vi "write1.vi"() -> ()   [LabVIEW 2020]
uses:
  TEST5/LabVIEW Example(8.6)/ControlCAN/ControlCAN.llb/Return Val.ctl
  TEST4/LabVIEW Example(8.6)/ControlCAN/ControlCAN.llb/VCI_CAN_OBJ.ctl
  TEST4/LabVIEW Example(8.6)/ControlCAN/ControlCAN.llb/DevType.ctl
  TEST1/ControlCAN/ControlCAN.llb/VCI_INIT_CONFIG.ctl
  TEST1/ControlCAN/ControlCAN.llb/InitFlag.ctl
  TEST1/ControlCAN/ControlCAN.llb/Fliter.ctl
  TEST1/ControlCAN/ControlCAN.llb/Mode.ctl
  TEST4/LabVIEW Example(8.6)/ControlCAN/ControlCAN.lvlib
panel:
  in  "Len 4":u32=2500 caption="Len(2500)"
  out "Recieve 4":T1[](array[typedef])
  in  "Len 3":u32=2500 caption="Len(2500)"
  out "Recieve 3":T1[](array[typedef])
  in  "Len 2":u32=2500 caption="Len(2500)"
  out "Recieve 2":T1[](array[typedef])
  out "字符串 2":string
  in  "Data 6":string="00 01 02 03 04 05 06 07"
  out "Recieve":T1[](array[typedef])
  in  "Len":u32=2500 caption="Len(2500)"
  in  "选项卡控件":T2(tab)
  in  "位置环KdSet":bool
  in  "位置环的kdread":bool
  in  "位置环kd的值":i32=1000
  in  "位置环KiSet":bool
  in  "位置环的kiread":bool
  in  "ki的值":i32=1000
  in  "kpset":bool
  in  "kpread":bool
  in  "实际位置":bool
  in  "设定位置":bool
  in  "转向电机使能":bool
  in  "停止":bool
  in  "ID":u32=291 format="0x%x"
  in  "转向电机使能：":i32=1000
  in  "位置环：\n     设定位置 2":i32=1000
  in  "kp的值":i32=1000
  out "实际位置":i16
  out "Return Val 2":T3=1 items=["OK"=1, "ERROR1"=0, "ERROR2"=-1]
  # "角度"
  # "角度"
  # "位置环id"
  # "Kp"
  # "Ki"
  # "Kd"
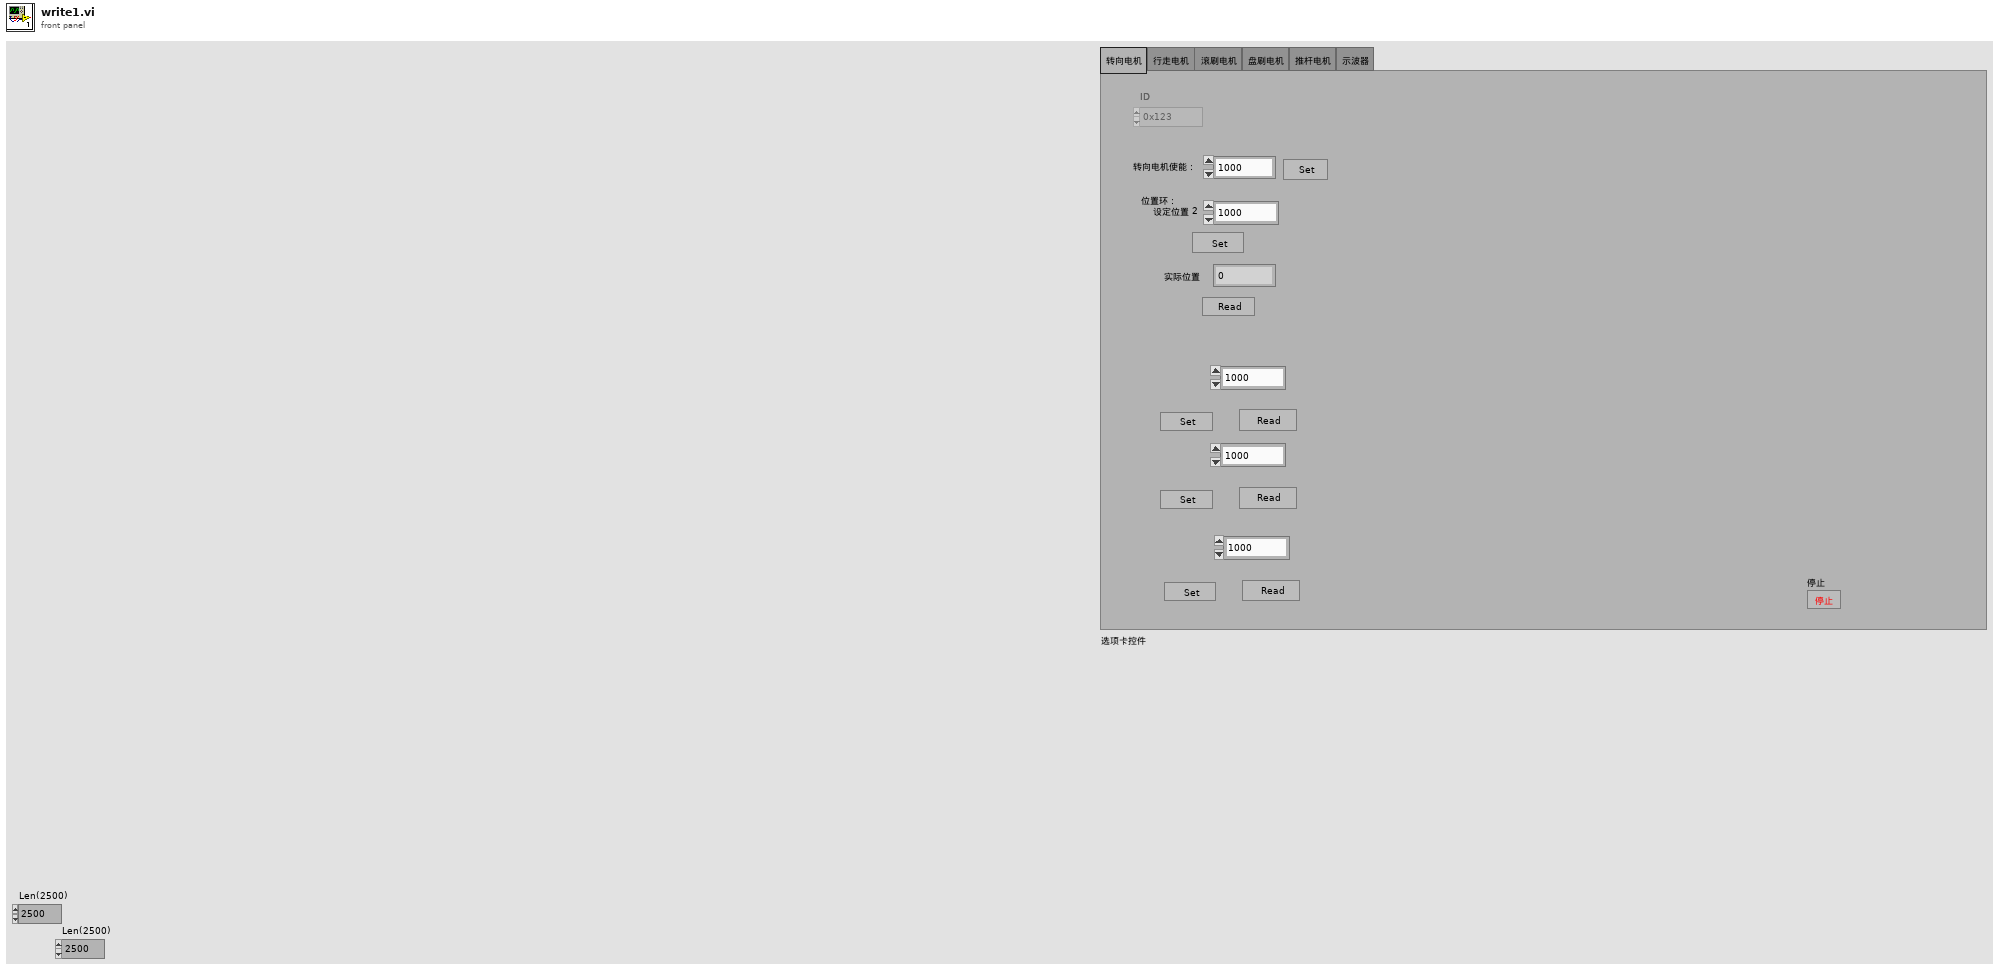
[diagram p1: front panel]
types:
  T1 = typedef "ControlCAN.lvlib/VCI_CAN_OBJ.ctl" = cluster{"ID":u32, "TimeStamp":u32, "TimeFlag":u8, "SendType":u8, "RemoteFlag":u8, "ExternFlag":u8, "DataLen":u8, "Data":u8[], "Reserved":u8[]}
  T2 = enum32{"转向电机", "行走电机", "滚刷电机", "盘刷电机", "推杆电机", "示波器"}
  T3 = typedef "ControlCAN.lvlib/Return Val.ctl" = i32
  T4 = typedef "ControlCAN.lvlib/VCI_INIT_CONFIG.ctl" = cluster{"AccCode":u32, "AccMask":u32, "InitFlag":T5, "Fliter":T6, "Timing0":u8, "Timing1":u8, "Mode":T7}
  T5 = typedef "ControlCAN.lvlib/InitFlag.ctl" = u32
  T6 = typedef "ControlCAN.lvlib/Fliter.ctl" = u8
  T7 = typedef "ControlCAN.lvlib/Mode.ctl" = u8
  T8 = typedef "ControlCAN.lvlib/DevType.ctl" = u32
  T9 = cluster{"Recieve 2[0]":T1, "Recieve 2[1]":T1, "Recieve 2[2]":T1, "Recieve 2[3]":T1, "Recieve 2[4]":T1, "Recieve 2[5]":T1, "Recieve 2[6]":T1, "Recieve 2[7]":T1, "Recieve 2[8]":T1}
  T10 = cluster{"Data[0]":u8, "Data[1]":u8, "Data[2]":u8, "Data[3]":u8, "Data[4]":u8, "Data[5]":u8, "Data[6]":u8, "Data[7]":u8, "Data[8]":u8}
  T11 = cluster{"Recieve[0]":T1, "Recieve[1]":T1, "Recieve[2]":T1, "Recieve[3]":T1, "Recieve[4]":T1, "Recieve[5]":T1, "Recieve[6]":T1, "Recieve[7]":T1, "Recieve[8]":T1}
  T12 = cluster{"Recieve 3[0]":T1, "Recieve 3[1]":T1, "Recieve 3[2]":T1, "Recieve 3[3]":T1, "Recieve 3[4]":T1, "Recieve 3[5]":T1, "Recieve 3[6]":T1, "Recieve 3[7]":T1, "Recieve 3[8]":T1}
  T13 = cluster{"Recieve 4[0]":T1, "Recieve 4[1]":T1, "Recieve 4[2]":T1, "Recieve 4[3]":T1, "Recieve 4[4]":T1, "Recieve 4[5]":T1, "Recieve 4[6]":T1, "Recieve 4[7]":T1, "Recieve 4[8]":T1}
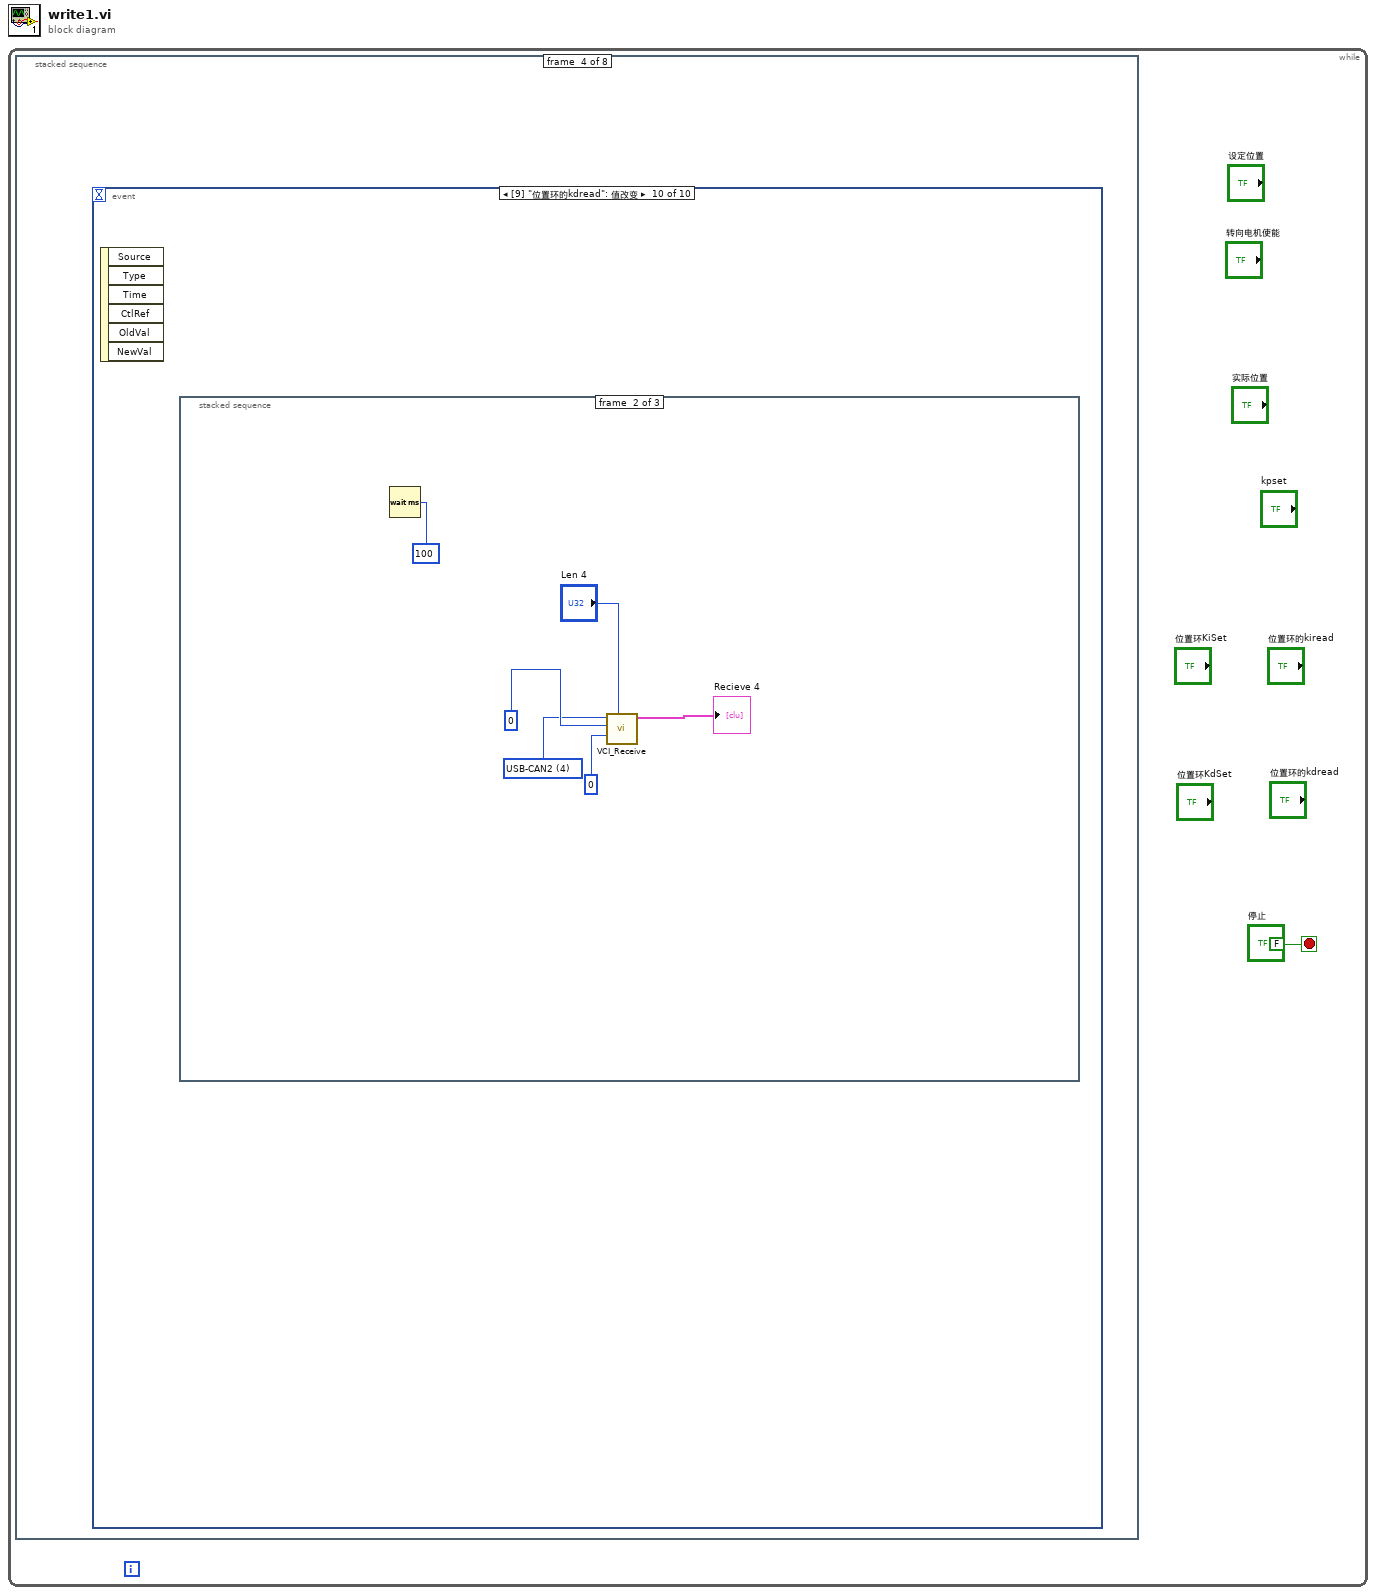
[diagram p0: block diagram]
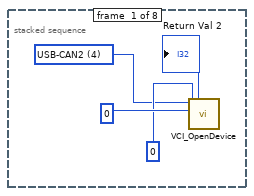
[diagram p2: hidden frame]
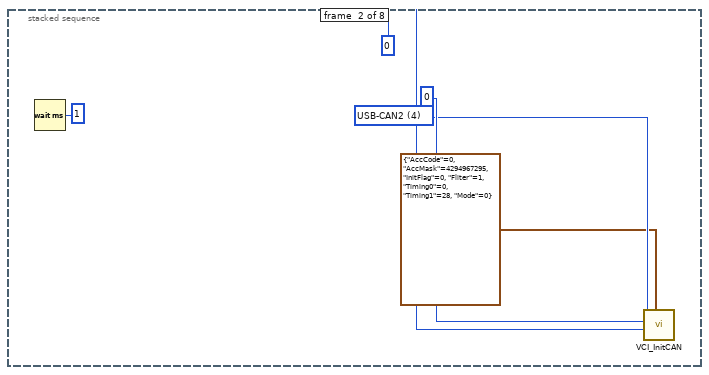
[diagram p3: hidden frame]
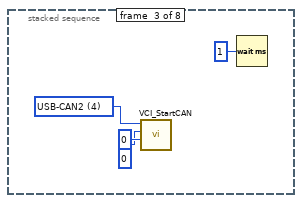
[diagram p4: hidden frame]
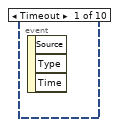
[diagram p5: hidden frame]
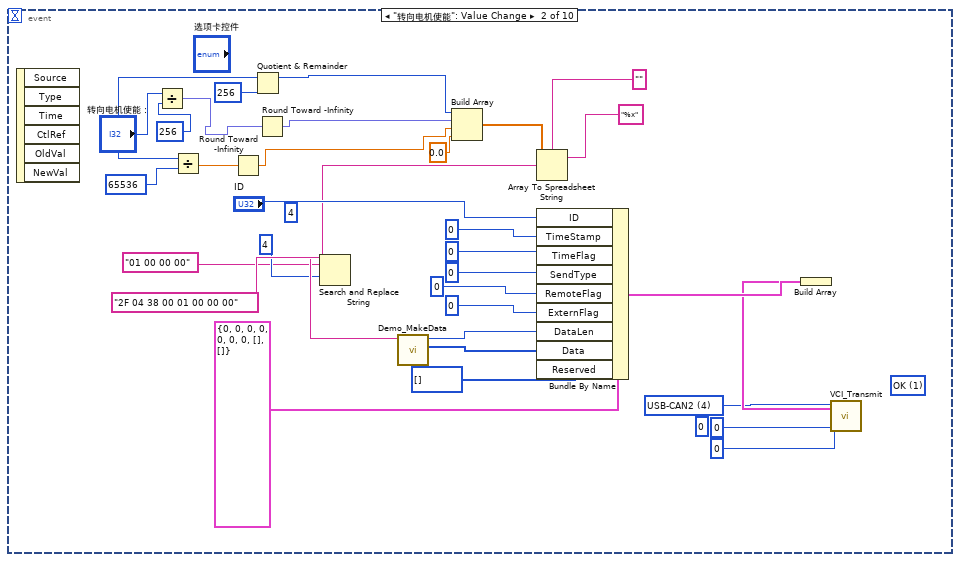
[diagram p6: hidden frame]
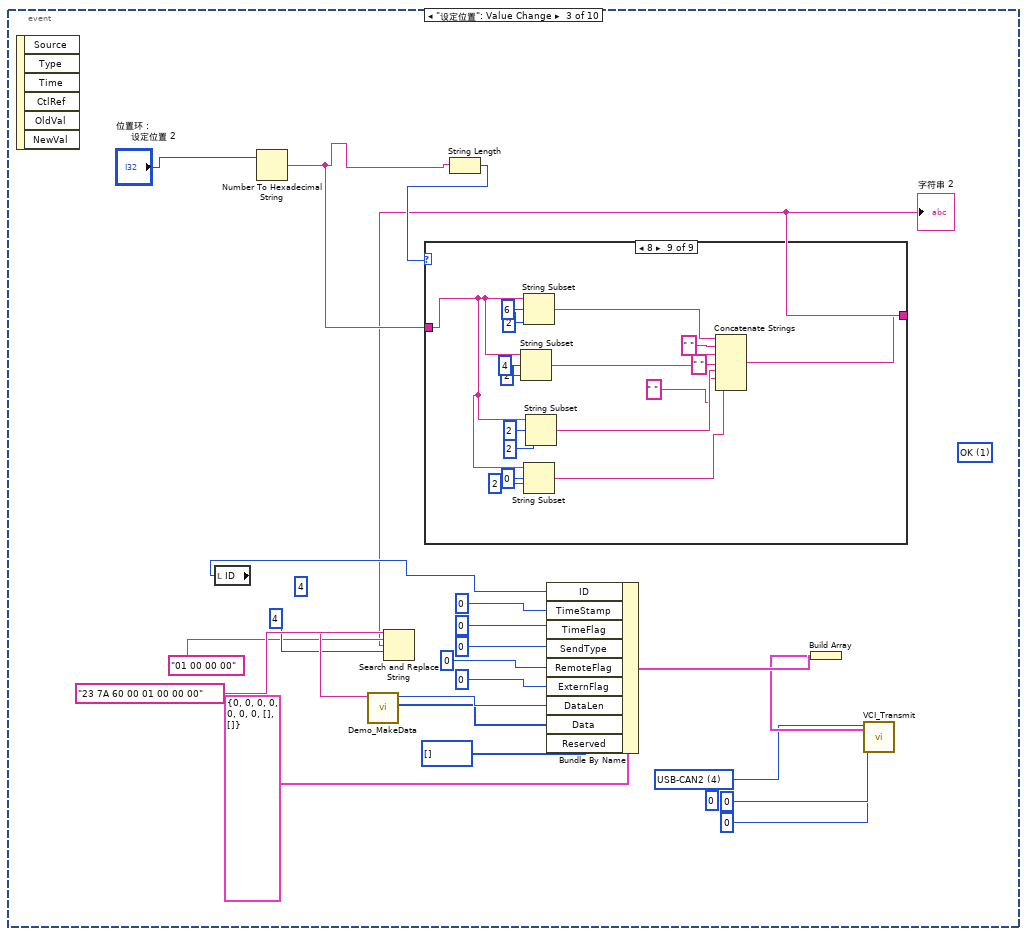
[diagram p7: hidden frame]
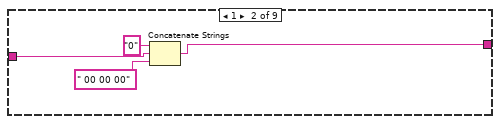
[diagram p9: hidden frame]
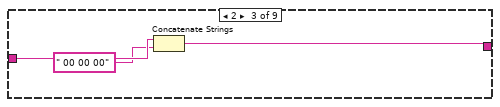
[diagram p10: hidden frame]
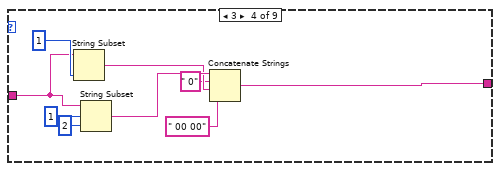
[diagram p11: hidden frame]
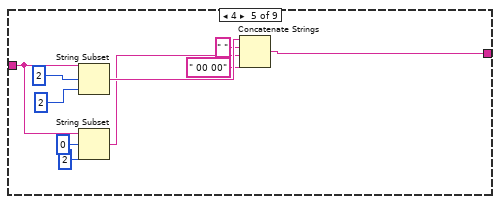
[diagram p12: hidden frame]
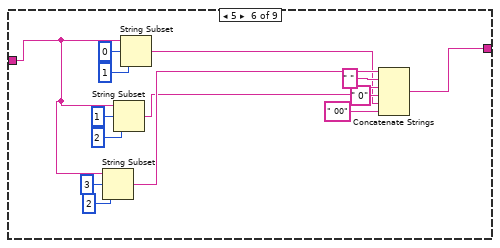
[diagram p13: hidden frame]
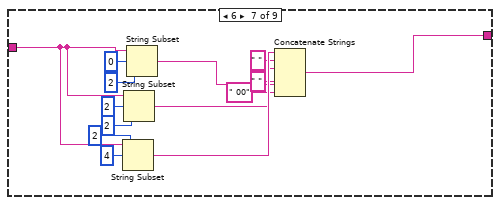
[diagram p14: hidden frame]
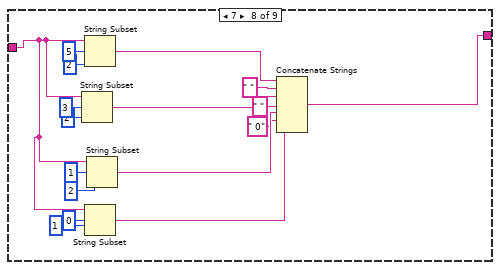
[diagram p15: hidden frame]
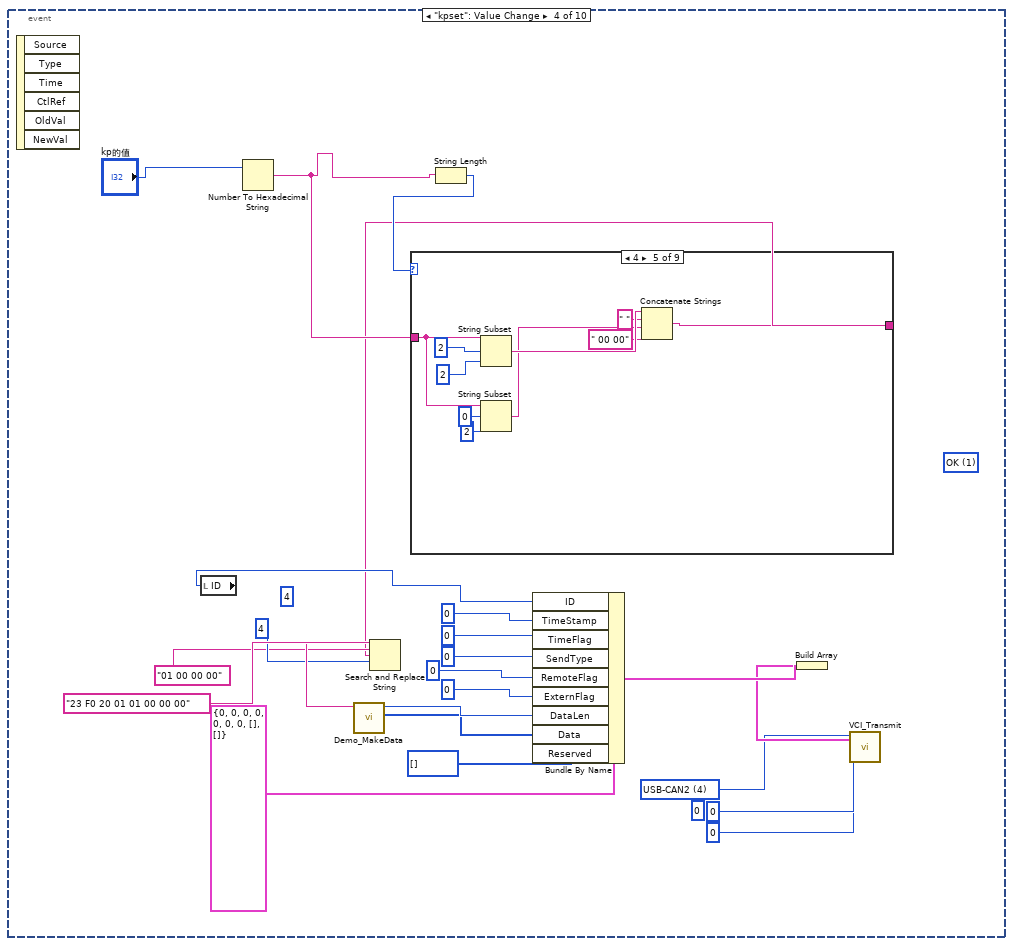
[diagram p16: hidden frame]
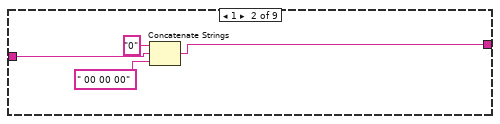
[diagram p18: hidden frame]
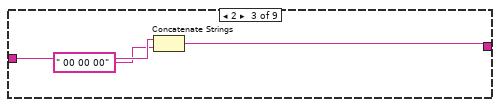
[diagram p19: hidden frame]
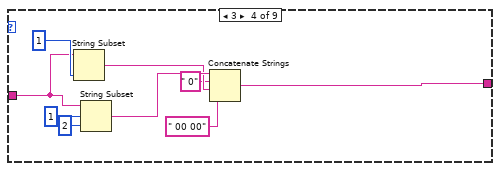
[diagram p20: hidden frame]
diagram:
  n1 = while {
    stop <- FALSE stop-if-true
    n2 = stacked-sequence {
      frame #0 {
        w2 = T8 4 items=["USB-CAN"=3, "USB-CAN2"=4] ("DevType")
        n3 = call "VCI_OpenDevice.vi"("Reserved"=u32 0, "DevIndex"=u32 0, "DevType"=w2) -> ("Return Val"=→"Return Val 2":T3)  [unwired: 7 in, 1 out]
      }
      frame #1 {
        w8 = T8 4 items=["USB-CAN"=3, "USB-CAN2"=4] ("DevType")
        n4 = Wait (ms)(milliseconds to wait=u32 1 ("等待时间（毫秒）")) -> ()  [unwired: 1 out]
        n5 = call "VCI_InitCAN.vi"("VCI_INIT_CONFIG"=T4 {"AccCode"=0, "AccMask"=4294967295, "InitFlag"=0, "Fliter"=1, "Timing0"=0, "Timing1"=28, "Mode"=0}, "CANIndex"=u32 0, "DevIndex"=u32 0, "DevType"=w8) -> ()  [unwired: 6 in, 2 out]
      }
      frame #2 {
        w12 = T8 4 items=["USB-CAN"=3, "USB-CAN2"=4] ("DevType")
        n6 = call "VCI_StartCAN.vi"("CANIndex"=u32 0, "DevIndex"=u32 0, "DevType"=w12) -> ()  [unwired: 7 in, 2 out]
        n7 = Wait (ms)(milliseconds to wait=u32 1 ("等待时间（毫秒）")) -> ()  [unwired: 1 out]
      }
      frame #3 {
        n8 = event shown="[9] \"位置环的kdread\": 值改变" {
          selector: _ -> [_ _ _ _ _ _ _ _ _ _]
          dyn-events: _ -> [_ _ _ _ _ _ _ _ _ _]
          timeout: _ -> [_ _ _ _ _ _ _ _ _ _]
          event Timeout {
            n9 = event-data() -> ()  [unwired: 1 in, 3 out]
          }
          event "转向电机使能": Value Change {
            (unwired) 4 ("替换数量")
            (unwired) T3 1 items=["OK"=1, "ERROR1"=0, "ERROR2"=-1] ("Return Val")
            (unwired) u32 0 ("CANIndex")
            w36 = T8 4 items=["USB-CAN"=3, "USB-CAN2"=4] ("DevType")
            n10 = event-data() -> ()  [unwired: 1 in, 6 out]
            n11 = Divide ("除")(x="转向电机使能：", y=256) -> (x/y=w20:fxp<+/-,32,16>)
            n12 = Divide(x="转向电机使能：", y=65536) -> (x/y=w17:dbl)
            n13 = Round Toward -Infinity(1:w17) -> (0:w16:dbl)
            n14 = Quotient & Remainder(x="转向电机使能：", y=256) -> (x-y*floor(x/y)=w19:i32)  [unwired: 1 out]
            n15 = Round Toward -Infinity(1:w20) -> (0:w18:fxp<+/-,16,16>)
            n16 = Build Array(w19, w18, w16, 0.0 ("元素")) -> (w25:dbl[])
            n17 = Array To Spreadsheet String(delimiter (Tab)="" ("分隔符(Tab)"), array=w25, 3:"%x" ("格式字符串")) -> (spreadsheet string=w26:string)
            n18 = Search and Replace String(input string="2F 04 38 00 01 00 00 00" ("Data 2"), search string="01 00 00 00" ("Data 4"), replace string=w26, offset=4 ("偏移量(0)")) -> (result string=w31:string)  [unwired: 4 in, 3 out]
            n19 = call "Demo_MakeData.vi"("DataString"=w31) -> ("Data"=w43:u8[], "DataLen"=w44:u8)  [unwired: 9 out]
            n20 = Bundle By Name(cluster=T1 {"ID"=0, "TimeStamp"=0, "TimeFlag"=0, "SendType"=0, "RemoteFlag"=0, "ExternFlag"=0, "DataLen"=0, "Data"=[], "Reserved"=[]} ("Send"), "ID"="ID", "TimeStamp"=u32 0, "TimeFlag"=u8 0, "SendType"=u8 0, "RemoteFlag"=u8 0, "ExternFlag"=u8 0, "DataLen"=w44, "Data"=w43, "Reserved"=u8[] []) -> (w46:T1)
            n21 = Build Array(w46) -> (w45:T1[])
            n22 = call "VCI_Transmit.vi"("Buffer"=w45, "CANIndex"=u32 0, "DevIndex"=u32 0, "DevType"=w36) -> ()  [unwired: 6 in, 2 out]
          }
          event "设定位置": Value Change {
            (unwired) 4 ("替换数量")
            (unwired) T3 1 items=["OK"=1, "ERROR1"=0, "ERROR2"=-1] ("Return Val")
            (unwired) u32 0 ("CANIndex")
            w61 = T8 4 items=["USB-CAN"=3, "USB-CAN2"=4] ("DevType")
            n23 = event-data() -> ()  [unwired: 1 in, 6 out]
            n24 = local read "ID"() -> (w53:u32)
            n25 = Number To Hexadecimal String(2:"位置环：\n     设定位置 2") -> (0:w49:string)  [unwired: 1 in]
            n26 = String Length(string=w49) -> (length=w50:i32)
            n27 = case shown="8" w50 {
              tunnel: w49 -> [w71 w74 w77 w84 w93 w107 w120 w136 w146]
              tunnel: [w71 w73 w78 w79 w97 w104 w125 w126 w145] -> w48
              frame 0, Default {
              }
              frame 1 {
                n28 = Concatenate Strings("0" ("字符串"), w74, " 00 00 00" ("字符串")) -> (w73:string)
              }
              frame 2 {
                n29 = Concatenate Strings(w77, " 00 00 00" ("字符串")) -> (w78:string)
              }
              frame 3 {
                n30 = String Subset(string=w84, length (rest)=1 ("长度（剩余）")) -> (substring=w82:string)  [unwired: 1 in]
                n31 = String Subset(string=w84, offset (0)=1 ("偏移量(0)"), length (rest)=2 ("长度（剩余）")) -> (substring=w83:string)
                n32 = Concatenate Strings(w83, " 0" ("字符串"), w82, " 00 00" ("字符串")) -> (w79:string)
              }
              frame 4 {
                n33 = String Subset(string=w93, offset (0)=2 ("偏移量(0)"), length (rest)=2 ("长度（剩余）")) -> (substring=w94:string)
                n34 = String Subset(string=w93, offset (0)=0 ("偏移量(0)"), length (rest)=2 ("长度（剩余）")) -> (substring=w89:string)
                n35 = Concatenate Strings(w94, " " ("字符串"), w89, " 00 00" ("字符串")) -> (w97:string)
              }
              frame 5 {
                n36 = String Subset(string=w107, offset (0)=3 ("偏移量(0)"), length (rest)=2 ("长度（剩余）")) -> (substring=w103:string)
                n37 = String Subset(string=w107, offset (0)=1 ("偏移量(0)"), length (rest)=2 ("长度（剩余）")) -> (substring=w101:string)
                n38 = String Subset(string=w107, offset (0)=0 ("偏移量(0)"), length (rest)=1 ("长度（剩余）")) -> (substring=w99:string)
                n39 = Concatenate Strings(w103, " " ("字符串"), w101, " 0" ("字符串"), w99, " 00" ("字符串")) -> (w104:string)
              }
              frame 6 {
                n40 = String Subset(string=w120, offset (0)=4 ("偏移量(0)"), length (rest)=2 ("长度（剩余）")) -> (substring=w117:string)
                n41 = String Subset(string=w120, offset (0)=2 ("偏移量(0)"), length (rest)=2 ("长度（剩余）")) -> (substring=w115:string)
                n42 = String Subset(string=w120, offset (0)=0 ("偏移量(0)"), length (rest)=2 ("长度（剩余）")) -> (substring=w113:string)
                n43 = Concatenate Strings(w117, " " ("字符串"), w115, " " ("字符串"), w113, " 00" ("字符串")) -> (w125:string)
              }
              frame 7 {
                n44 = String Subset(string=w136, offset (0)=3 ("偏移量(0)"), length (rest)=2 ("长度（剩余）")) -> (substring=w131:string)
                n45 = String Subset(string=w136, offset (0)=5 ("偏移量(0)"), length (rest)=2 ("长度（剩余）")) -> (substring=w133:string)
                n46 = String Subset(string=w136, offset (0)=0 ("偏移量(0)"), length (rest)=1 ("长度（剩余）")) -> (substring=w127:string)
                n47 = String Subset(string=w136, offset (0)=1 ("偏移量(0)"), length (rest)=2 ("长度（剩余）")) -> (substring=w129:string)
                n48 = Concatenate Strings(w133, " " ("字符串"), w131, " " ("字符串"), w129, " 0" ("字符串"), w127) -> (w126:string)
              }
              frame 8 {
                n49 = String Subset(string=w146, offset (0)=4 ("偏移量(0)"), length (rest)=2 ("长度（剩余）")) -> (substring=w149:string)
                n50 = String Subset(string=w146, offset (0)=6 ("偏移量(0)"), length (rest)=2 ("长度（剩余）")) -> (substring=w151:string)
                n51 = String Subset(string=w146, offset (0)=0 ("偏移量(0)"), length (rest)=2 ("长度（剩余）")) -> (substring=w143:string)
                n52 = String Subset(string=w146, offset (0)=2 ("偏移量(0)"), length (rest)=2 ("长度（剩余）")) -> (substring=w147:string)
                n53 = Concatenate Strings(w151, " " ("字符串"), w149, " " ("字符串"), w147, " " ("字符串"), w143) -> (w145:string)
              }
            }
            "字符串 2" <- w48
            n54 = Search and Replace String(input string="23 7A 60 00 01 00 00 00" ("Data 3"), search string="01 00 00 00" ("Data 5"), replace string=w48, offset=4 ("偏移量(0)")) -> (result string=w56:string)  [unwired: 4 in, 3 out]
            n55 = call "Demo_MakeData.vi"("DataString"=w56) -> ("Data"=w52:u8[], "DataLen"=w67:u8)  [unwired: 9 out]
            n56 = Bundle By Name(cluster=T1 {"ID"=0, "TimeStamp"=0, "TimeFlag"=0, "SendType"=0, "RemoteFlag"=0, "ExternFlag"=0, "DataLen"=0, "Data"=[], "Reserved"=[]} ("Send"), "ID"=w53, "TimeStamp"=u32 0, "TimeFlag"=u8 0, "SendType"=u8 0, "RemoteFlag"=u8 0, "ExternFlag"=u8 0, "DataLen"=w67, "Data"=w52, "Reserved"=u8[] []) -> (w69:T1)
            n57 = Build Array(w69) -> (w68:T1[])
            n58 = call "VCI_Transmit.vi"("Buffer"=w68, "CANIndex"=u32 0, "DevIndex"=u32 0, "DevType"=w61) -> ()  [unwired: 6 in, 2 out]
          }
          event "kpset": Value Change {
            (unwired) 4 ("替换数量")
            (unwired) T3 1 items=["OK"=1, "ERROR1"=0, "ERROR2"=-1] ("Return Val")
            (unwired) u32 0 ("CANIndex")
            w173 = T8 4 items=["USB-CAN"=3, "USB-CAN2"=4] ("DevType")
            n59 = event-data() -> ()  [unwired: 1 in, 6 out]
            n60 = local read "ID"() -> (w165:u32)
            n61 = Number To Hexadecimal String(2:"kp的值") -> (0:w162:string)  [unwired: 1 in]
            n62 = String Length(string=w162) -> (length=w163:i32)
            n63 = case shown="4" w163 {
              tunnel: w162 -> [w183 w186 w189 w196 w205 w219 w232 w248 w258]
              tunnel: [w183 w185 w190 w191 w209 w216 w237 w238 w257] -> w160
              frame 0, Default {
              }
              frame 1 {
                n64 = Concatenate Strings("0" ("字符串"), w186, " 00 00 00" ("字符串")) -> (w185:string)
              }
              frame 2 {
                n65 = Concatenate Strings(w189, " 00 00 00" ("字符串")) -> (w190:string)
              }
              frame 3 {
                n66 = String Subset(string=w196, length (rest)=1 ("长度（剩余）")) -> (substring=w194:string)  [unwired: 1 in]
                n67 = String Subset(string=w196, offset (0)=1 ("偏移量(0)"), length (rest)=2 ("长度（剩余）")) -> (substring=w195:string)
                n68 = Concatenate Strings(w195, " 0" ("字符串"), w194, " 00 00" ("字符串")) -> (w191:string)
              }
              frame 4 {
                n69 = String Subset(string=w205, offset (0)=2 ("偏移量(0)"), length (rest)=2 ("长度（剩余）")) -> (substring=w206:string)
                n70 = String Subset(string=w205, offset (0)=0 ("偏移量(0)"), length (rest)=2 ("长度（剩余）")) -> (substring=w201:string)
                n71 = Concatenate Strings(w206, " " ("字符串"), w201, " 00 00" ("字符串")) -> (w209:string)
              }
              frame 5 {
                n72 = String Subset(string=w219, offset (0)=3 ("偏移量(0)"), length (rest)=2 ("长度（剩余）")) -> (substring=w215:string)
                n73 = String Subset(string=w219, offset (0)=1 ("偏移量(0)"), length (rest)=2 ("长度（剩余）")) -> (substring=w213:string)
                n74 = String Subset(string=w219, offset (0)=0 ("偏移量(0)"), length (rest)=1 ("长度（剩余）")) -> (substring=w211:string)
                n75 = Concatenate Strings(w215, " " ("字符串"), w213, " 0" ("字符串"), w211, " 00" ("字符串")) -> (w216:string)
              }
              frame 6 {
                n76 = String Subset(string=w232, offset (0)=4 ("偏移量(0)"), length (rest)=2 ("长度（剩余）")) -> (substring=w229:string)
                n77 = String Subset(string=w232, offset (0)=2 ("偏移量(0)"), length (rest)=2 ("长度（剩余）")) -> (substring=w227:string)
                n78 = String Subset(string=w232, offset (0)=0 ("偏移量(0)"), length (rest)=2 ("长度（剩余）")) -> (substring=w225:string)
                n79 = Concatenate Strings(w229, " " ("字符串"), w227, " " ("字符串"), w225, " 00" ("字符串")) -> (w237:string)
              }
              frame 7 {
                n80 = String Subset(string=w248, offset (0)=3 ("偏移量(0)"), length (rest)=2 ("长度（剩余）")) -> (substring=w243:string)
                n81 = String Subset(string=w248, offset (0)=5 ("偏移量(0)"), length (rest)=2 ("长度（剩余）")) -> (substring=w245:string)
                n82 = String Subset(string=w248, offset (0)=0 ("偏移量(0)"), length (rest)=1 ("长度（剩余）")) -> (substring=w239:string)
                n83 = String Subset(string=w248, offset (0)=1 ("偏移量(0)"), length (rest)=2 ("长度（剩余）")) -> (substring=w241:string)
                n84 = Concatenate Strings(w245, " " ("字符串"), w243, " " ("字符串"), w241, " 0" ("字符串"), w239) -> (w238:string)
              }
              frame 8 {
                n85 = String Subset(string=w258, offset (0)=4 ("偏移量(0)"), length (rest)=2 ("长度（剩余）")) -> (substring=w261:string)
                n86 = String Subset(string=w258, offset (0)=6 ("偏移量(0)"), length (rest)=2 ("长度（剩余）")) -> (substring=w263:string)
                n87 = String Subset(string=w258, offset (0)=0 ("偏移量(0)"), length (rest)=2 ("长度（剩余）")) -> (substring=w255:string)
                n88 = String Subset(string=w258, offset (0)=2 ("偏移量(0)"), length (rest)=2 ("长度（剩余）")) -> (substring=w259:string)
                n89 = Concatenate Strings(w263, " " ("字符串"), w261, " " ("字符串"), w259, " " ("字符串"), w255) -> (w257:string)
              }
            }
            n90 = Search and Replace String(input string="23 F0 20 01 01 00 00 00" ("Data 3"), search string="01 00 00 00" ("Data 5"), replace string=w160, offset=4 ("偏移量(0)")) -> (result string=w168:string)  [unwired: 4 in, 3 out]
            n91 = call "Demo_MakeData.vi"("DataString"=w168) -> ("Data"=w164:u8[], "DataLen"=w179:u8)  [unwired: 9 out]
            n92 = Bundle By Name(cluster=T1 {"ID"=0, "TimeStamp"=0, "TimeFlag"=0, "SendType"=0, "RemoteFlag"=0, "ExternFlag"=0, "DataLen"=0, "Data"=[], "Reserved"=[]} ("Send"), "ID"=w165, "TimeStamp"=u32 0, "TimeFlag"=u8 0, "SendType"=u8 0, "RemoteFlag"=u8 0, "ExternFlag"=u8 0, "DataLen"=w179, "Data"=w164, "Reserved"=u8[] []) -> (w181:T1)
            n93 = Build Array(w181) -> (w180:T1[])
            n94 = call "VCI_Transmit.vi"("Buffer"=w180, "CANIndex"=u32 0, "DevIndex"=u32 0, "DevType"=w173) -> ()  [unwired: 6 in, 2 out]
          }
          event "kpread": Value Change {
            n95 = event-data() -> ()  [unwired: 1 in, 6 out]
            n96 = stacked-sequence {
              frame #0 {
                (unwired) u32 0 ("CANIndex")
                w278 = T8 4 items=["USB-CAN"=3, "USB-CAN2"=4] ("DevType")
                n97 = local read "ID"() -> (w273:u32)
                n98 = call "Demo_MakeData.vi"("DataString"="40 F0 20 01 00 00 00 00" ("Data 7")) -> ("Data"=w284:u8[], "DataLen"=w285:u8)  [unwired: 9 out]
                n99 = Bundle By Name(cluster=T1 {"ID"=0, "TimeStamp"=0, "TimeFlag"=0, "SendType"=0, "RemoteFlag"=0, "ExternFlag"=0, "DataLen"=0, "Data"=[], "Reserved"=[]} ("Send"), "ID"=w273, "TimeStamp"=u32 0, "TimeFlag"=u8 0, "SendType"=u8 0, "RemoteFlag"=u8 0, "ExternFlag"=u8 0, "DataLen"=w285, "Data"=w284, "Reserved"=u8[] []) -> (w287:T1)
                n100 = Build Array(w287) -> (w286:T1[])
                n101 = call "VCI_Transmit.vi"("Buffer"=w286, "CANIndex"=u32 0, "DevIndex"=u32 0, "DevType"=w278) -> ()  [unwired: 6 in, 2 out]
              }
              frame #1 {
                w288 = T8 4 items=["USB-CAN"=3, "USB-CAN2"=4] ("DevType")
                n102 = Wait (ms)(milliseconds to wait=u32 100 ("等待时间（毫秒）")) -> ()  [unwired: 1 out]
                n103 = call "VCI_Receive.vi"("Len"="Len 2", "CANIndex"=u32 0, "DevIndex"=u32 0, "DevType"=w288) -> ("Recieve"=→"Recieve 2":T1[])  [unwired: 6 in, 1 out]
              }
              frame #2 {
                n104 = local read "Recieve 2"() -> (w310:T1[])
                n105 = Array To Cluster(array=w310) -> (cluster=w309:T9)
                n106 = Unbundle By Name(w309) -> ("Recieve 2[0].Data"=w308:u8[])
                n107 = Array To Cluster(array=w308) -> (cluster=w307:T10)
                n108 = Unbundle By Name(w307) -> ("Data[6]"=w302:u8)
                n109 = Unbundle By Name(w307) -> ("Data[7]"=w301:u8)
                n110 = Unbundle By Name(w307) -> ("Data[5]"=w306:u8)
                n111 = Unbundle By Name(w307) -> ("Data[4]"=w303:u8)
                n112 = Multiply(x=w301, y=16777216) -> (x*y=w297:i32)
                n113 = Multiply(x=w302, y=65536) -> (x*y=w298:i32)
                n114 = Multiply(x=w306, y=256.0) -> (x*y=w304:dbl)
                n115 = Add(x=w303, y=w304) -> (x+y=w296:dbl)
                n116 = Add(x=w298, y=w297) -> (x+y=w295:i32)
                n117 = Add(x=w296, y=w295) -> (x+y=→"实际位置":dbl)
              }
            }
          }
          event "实际位置": Value Change {
            n118 = event-data() -> ()  [unwired: 1 in, 6 out]
            n119 = stacked-sequence {
              frame #0 {
                (unwired) u32 0 ("CANIndex")
                w317 = T8 4 items=["USB-CAN"=3, "USB-CAN2"=4] ("DevType")
                n120 = local read "ID"() -> (w312:u32)
                n121 = call "Demo_MakeData.vi"("DataString"="Data 6") -> ("Data"=w323:u8[], "DataLen"=w324:u8)  [unwired: 9 out]
                n122 = Bundle By Name(cluster=T1 {"ID"=0, "TimeStamp"=0, "TimeFlag"=0, "SendType"=0, "RemoteFlag"=0, "ExternFlag"=0, "DataLen"=0, "Data"=[], "Reserved"=[]} ("Send"), "ID"=w312, "TimeStamp"=u32 0, "TimeFlag"=u8 0, "SendType"=u8 0, "RemoteFlag"=u8 0, "ExternFlag"=u8 0, "DataLen"=w324, "Data"=w323, "Reserved"=u8[] []) -> (w326:T1)
                n123 = Build Array(w326) -> (w325:T1[])
                n124 = call "VCI_Transmit.vi"("Buffer"=w325, "CANIndex"=u32 0, "DevIndex"=u32 0, "DevType"=w317) -> ()  [unwired: 6 in, 2 out]
              }
              frame #1 {
                w327 = T8 4 items=["USB-CAN"=3, "USB-CAN2"=4] ("DevType")
                n125 = Wait (ms)(milliseconds to wait=u32 100 ("等待时间（毫秒）")) -> ()  [unwired: 1 out]
                n126 = call "VCI_Receive.vi"("Len"="Len", "CANIndex"=u32 0, "DevIndex"=u32 0, "DevType"=w327) -> ("Recieve"=→"Recieve":T1[])  [unwired: 6 in, 1 out]
              }
              frame #2 {
                n127 = local read "Recieve"() -> (w349:T1[])
                n128 = Array To Cluster(array=w349) -> (cluster=w348:T11)
                n129 = Unbundle By Name(w348) -> ("Recieve[0].Data"=w347:u8[])
                n130 = Array To Cluster(array=w347) -> (cluster=w346:T10)
                n131 = Unbundle By Name(w346) -> ("Data[6]"=w341:u8)
                n132 = Unbundle By Name(w346) -> ("Data[7]"=w340:u8)
                n133 = Unbundle By Name(w346) -> ("Data[5]"=w345:u8)
                n134 = Unbundle By Name(w346) -> ("Data[4]"=w342:u8)
                n135 = Multiply(x=w340, y=16777216) -> (x*y=w336:i32)
                n136 = Multiply(x=w341, y=65536) -> (x*y=w337:i32)
                n137 = Multiply(x=w345, y=256.0) -> (x*y=w343:dbl)
                n138 = Add(x=w342, y=w343) -> (x+y=w335:dbl)
                n139 = Add(x=w337, y=w336) -> (x+y=w334:i32)
                n140 = Add(x=w335, y=w334) -> (x+y=w333:dbl)
                n141 = local write "kp的值"(w333) -> ()
              }
            }
          }
          event "位置环KiSet": Value Change {
            (unwired) 4 ("替换数量")
            (unwired) u32 0 ("CANIndex")
            w363 = T8 4 items=["USB-CAN"=3, "USB-CAN2"=4] ("DevType")
            n142 = event-data() -> ()  [unwired: 1 in, 6 out]
            n143 = local read "ID"() -> (w355:u32)
            n144 = Number To Hexadecimal String(2:"ki的值") -> (0:w352:string)  [unwired: 1 in]
            n145 = String Length(string=w352) -> (length=w353:i32)
            n146 = case shown="4" w353 {
              tunnel: w352 -> [w373 w376 w379 w386 w395 w409 w422 w438 w448]
              tunnel: [w373 w375 w380 w381 w399 w406 w427 w428 w447] -> w351
              frame 0, Default {
              }
              frame 1 {
                n147 = Concatenate Strings("0" ("字符串"), w376, " 00 00 00" ("字符串")) -> (w375:string)
              }
              frame 2 {
                n148 = Concatenate Strings(w379, " 00 00 00" ("字符串")) -> (w380:string)
              }
              frame 3 {
                n149 = String Subset(string=w386, length (rest)=1 ("长度（剩余）")) -> (substring=w384:string)  [unwired: 1 in]
                n150 = String Subset(string=w386, offset (0)=1 ("偏移量(0)"), length (rest)=2 ("长度（剩余）")) -> (substring=w385:string)
                n151 = Concatenate Strings(w385, " 0" ("字符串"), w384, " 00 00" ("字符串")) -> (w381:string)
              }
              frame 4 {
                n152 = String Subset(string=w395, offset (0)=2 ("偏移量(0)"), length (rest)=2 ("长度（剩余）")) -> (substring=w396:string)
                n153 = String Subset(string=w395, offset (0)=0 ("偏移量(0)"), length (rest)=2 ("长度（剩余）")) -> (substring=w391:string)
                n154 = Concatenate Strings(w396, " " ("字符串"), w391, " 00 00" ("字符串")) -> (w399:string)
              }
              frame 5 {
                n155 = String Subset(string=w409, offset (0)=3 ("偏移量(0)"), length (rest)=2 ("长度（剩余）")) -> (substring=w405:string)
                n156 = String Subset(string=w409, offset (0)=1 ("偏移量(0)"), length (rest)=2 ("长度（剩余）")) -> (substring=w403:string)
                n157 = String Subset(string=w409, offset (0)=0 ("偏移量(0)"), length (rest)=1 ("长度（剩余）")) -> (substring=w401:string)
                n158 = Concatenate Strings(w405, " " ("字符串"), w403, " 0" ("字符串"), w401, " 00" ("字符串")) -> (w406:string)
              }
              frame 6 {
                n159 = String Subset(string=w422, offset (0)=4 ("偏移量(0)"), length (rest)=2 ("长度（剩余）")) -> (substring=w419:string)
                n160 = String Subset(string=w422, offset (0)=2 ("偏移量(0)"), length (rest)=2 ("长度（剩余）")) -> (substring=w417:string)
                n161 = String Subset(string=w422, offset (0)=0 ("偏移量(0)"), length (rest)=2 ("长度（剩余）")) -> (substring=w415:string)
                n162 = Concatenate Strings(w419, " " ("字符串"), w417, " " ("字符串"), w415, " 00" ("字符串")) -> (w427:string)
              }
              frame 7 {
                n163 = String Subset(string=w438, offset (0)=3 ("偏移量(0)"), length (rest)=2 ("长度（剩余）")) -> (substring=w433:string)
                n164 = String Subset(string=w438, offset (0)=5 ("偏移量(0)"), length (rest)=2 ("长度（剩余）")) -> (substring=w435:string)
                n165 = String Subset(string=w438, offset (0)=0 ("偏移量(0)"), length (rest)=1 ("长度（剩余）")) -> (substring=w429:string)
                n166 = String Subset(string=w438, offset (0)=1 ("偏移量(0)"), length (rest)=2 ("长度（剩余）")) -> (substring=w431:string)
                n167 = Concatenate Strings(w435, " " ("字符串"), w433, " " ("字符串"), w431, " 0" ("字符串"), w429) -> (w428:string)
              }
              frame 8 {
                n168 = String Subset(string=w448, offset (0)=4 ("偏移量(0)"), length (rest)=2 ("长度（剩余）")) -> (substring=w451:string)
                n169 = String Subset(string=w448, offset (0)=6 ("偏移量(0)"), length (rest)=2 ("长度（剩余）")) -> (substring=w453:string)
                n170 = String Subset(string=w448, offset (0)=0 ("偏移量(0)"), length (rest)=2 ("长度（剩余）")) -> (substring=w445:string)
                n171 = String Subset(string=w448, offset (0)=2 ("偏移量(0)"), length (rest)=2 ("长度（剩余）")) -> (substring=w449:string)
                n172 = Concatenate Strings(w453, " " ("字符串"), w451, " " ("字符串"), w449, " " ("字符串"), w445) -> (w447:string)
              }
            }
            n173 = Search and Replace String(input string="23 F0 20 02 01 00 00 00" ("Data 3"), search string="01 00 00 00" ("Data 5"), replace string=w351, offset=4 ("偏移量(0)")) -> (result string=w358:string)  [unwired: 4 in, 3 out]
            n174 = call "Demo_MakeData.vi"("DataString"=w358) -> ("Data"=w354:u8[], "DataLen"=w369:u8)  [unwired: 9 out]
            n175 = Bundle By Name(cluster=T1 {"ID"=0, "TimeStamp"=0, "TimeFlag"=0, "SendType"=0, "RemoteFlag"=0, "ExternFlag"=0, "DataLen"=0, "Data"=[], "Reserved"=[]} ("Send"), "ID"=w355, "TimeStamp"=u32 0, "TimeFlag"=u8 0, "SendType"=u8 0, "RemoteFlag"=u8 0, "ExternFlag"=u8 0, "DataLen"=w369, "Data"=w354, "Reserved"=u8[] []) -> (w371:T1)
            n176 = Build Array(w371) -> (w370:T1[])
            n177 = call "VCI_Transmit.vi"("Buffer"=w370, "CANIndex"=u32 0, "DevIndex"=u32 0, "DevType"=w363) -> ()  [unwired: 6 in, 2 out]
          }
          event "位置环的kiread": Value Change {
            n178 = event-data() -> ()  [unwired: 1 in, 6 out]
            n179 = stacked-sequence {
              frame #0 {
                (unwired) u32 0 ("CANIndex")
                w468 = T8 4 items=["USB-CAN"=3, "USB-CAN2"=4] ("DevType")
                n180 = local read "ID"() -> (w463:u32)
                n181 = call "Demo_MakeData.vi"("DataString"="40 F0 20 02 00 00 00 00" ("Data 7")) -> ("Data"=w474:u8[], "DataLen"=w475:u8)  [unwired: 9 out]
                n182 = Bundle By Name(cluster=T1 {"ID"=0, "TimeStamp"=0, "TimeFlag"=0, "SendType"=0, "RemoteFlag"=0, "ExternFlag"=0, "DataLen"=0, "Data"=[], "Reserved"=[]} ("Send"), "ID"=w463, "TimeStamp"=u32 0, "TimeFlag"=u8 0, "SendType"=u8 0, "RemoteFlag"=u8 0, "ExternFlag"=u8 0, "DataLen"=w475, "Data"=w474, "Reserved"=u8[] []) -> (w477:T1)
                n183 = Build Array(w477) -> (w476:T1[])
                n184 = call "VCI_Transmit.vi"("Buffer"=w476, "CANIndex"=u32 0, "DevIndex"=u32 0, "DevType"=w468) -> ()  [unwired: 6 in, 2 out]
              }
              frame #1 {
                w478 = T8 4 items=["USB-CAN"=3, "USB-CAN2"=4] ("DevType")
                n185 = Wait (ms)(milliseconds to wait=u32 100 ("等待时间（毫秒）")) -> ()  [unwired: 1 out]
                n186 = call "VCI_Receive.vi"("Len"="Len 3", "CANIndex"=u32 0, "DevIndex"=u32 0, "DevType"=w478) -> ("Recieve"=→"Recieve 3":T1[])  [unwired: 6 in, 1 out]
              }
              frame #2 {
                n187 = local read "Recieve 3"() -> (w500:T1[])
                n188 = Array To Cluster(array=w500) -> (cluster=w499:T12)
                n189 = Unbundle By Name(w499) -> ("Recieve 3[0].Data"=w498:u8[])
                n190 = Array To Cluster(array=w498) -> (cluster=w497:T10)
                n191 = Unbundle By Name(w497) -> ("Data[6]"=w492:u8)
                n192 = Unbundle By Name(w497) -> ("Data[7]"=w491:u8)
                n193 = Unbundle By Name(w497) -> ("Data[5]"=w496:u8)
                n194 = Unbundle By Name(w497) -> ("Data[4]"=w493:u8)
                n195 = Multiply(x=w491, y=16777216) -> (x*y=w487:i32)
                n196 = Multiply(x=w492, y=65536) -> (x*y=w488:i32)
                n197 = Multiply(x=w496, y=256.0) -> (x*y=w494:dbl)
                n198 = Add(x=w493, y=w494) -> (x+y=w486:dbl)
                n199 = Add(x=w488, y=w487) -> (x+y=w485:i32)
                n200 = Add(x=w486, y=w485) -> (x+y=w484:dbl)
                n201 = local write "ki的值"(w484) -> ()
              }
            }
          }
          event "位置环KdSet": Value Change {
            (unwired) 4 ("替换数量")
            (unwired) u32 0 ("CANIndex")
            w514 = T8 4 items=["USB-CAN"=3, "USB-CAN2"=4] ("DevType")
            n202 = event-data() -> ()  [unwired: 1 in, 6 out]
            n203 = local read "ID"() -> (w506:u32)
            n204 = Number To Hexadecimal String(2:"位置环kd的值") -> (0:w503:string)  [unwired: 1 in]
            n205 = String Length(string=w503) -> (length=w504:i32)
            n206 = case shown="4" w504 {
              tunnel: w503 -> [w524 w527 w530 w537 w546 w560 w573 w589 w599]
              tunnel: [w524 w526 w531 w532 w550 w557 w578 w579 w598] -> w502
              frame 0, Default {
              }
              frame 1 {
                n207 = Concatenate Strings("0" ("字符串"), w527, " 00 00 00" ("字符串")) -> (w526:string)
              }
              frame 2 {
                n208 = Concatenate Strings(w530, " 00 00 00" ("字符串")) -> (w531:string)
              }
              frame 3 {
                n209 = String Subset(string=w537, length (rest)=1 ("长度（剩余）")) -> (substring=w535:string)  [unwired: 1 in]
                n210 = String Subset(string=w537, offset (0)=1 ("偏移量(0)"), length (rest)=2 ("长度（剩余）")) -> (substring=w536:string)
                n211 = Concatenate Strings(w536, " 0" ("字符串"), w535, " 00 00" ("字符串")) -> (w532:string)
              }
              frame 4 {
                n212 = String Subset(string=w546, offset (0)=2 ("偏移量(0)"), length (rest)=2 ("长度（剩余）")) -> (substring=w547:string)
                n213 = String Subset(string=w546, offset (0)=0 ("偏移量(0)"), length (rest)=2 ("长度（剩余）")) -> (substring=w542:string)
                n214 = Concatenate Strings(w547, " " ("字符串"), w542, " 00 00" ("字符串")) -> (w550:string)
              }
              frame 5 {
                n215 = String Subset(string=w560, offset (0)=3 ("偏移量(0)"), length (rest)=2 ("长度（剩余）")) -> (substring=w556:string)
                n216 = String Subset(string=w560, offset (0)=1 ("偏移量(0)"), length (rest)=2 ("长度（剩余）")) -> (substring=w554:string)
                n217 = String Subset(string=w560, offset (0)=0 ("偏移量(0)"), length (rest)=1 ("长度（剩余）")) -> (substring=w552:string)
                n218 = Concatenate Strings(w556, " " ("字符串"), w554, " 0" ("字符串"), w552, " 00" ("字符串")) -> (w557:string)
              }
              frame 6 {
                n219 = String Subset(string=w573, offset (0)=4 ("偏移量(0)"), length (rest)=2 ("长度（剩余）")) -> (substring=w570:string)
                n220 = String Subset(string=w573, offset (0)=2 ("偏移量(0)"), length (rest)=2 ("长度（剩余）")) -> (substring=w568:string)
                n221 = String Subset(string=w573, offset (0)=0 ("偏移量(0)"), length (rest)=2 ("长度（剩余）")) -> (substring=w566:string)
                n222 = Concatenate Strings(w570, " " ("字符串"), w568, " " ("字符串"), w566, " 00" ("字符串")) -> (w578:string)
              }
              frame 7 {
                n223 = String Subset(string=w589, offset (0)=3 ("偏移量(0)"), length (rest)=2 ("长度（剩余）")) -> (substring=w584:string)
                n224 = String Subset(string=w589, offset (0)=5 ("偏移量(0)"), length (rest)=2 ("长度（剩余）")) -> (substring=w586:string)
                n225 = String Subset(string=w589, offset (0)=0 ("偏移量(0)"), length (rest)=1 ("长度（剩余）")) -> (substring=w580:string)
                n226 = String Subset(string=w589, offset (0)=1 ("偏移量(0)"), length (rest)=2 ("长度（剩余）")) -> (substring=w582:string)
                n227 = Concatenate Strings(w586, " " ("字符串"), w584, " " ("字符串"), w582, " 0" ("字符串"), w580) -> (w579:string)
              }
              frame 8 {
                n228 = String Subset(string=w599, offset (0)=4 ("偏移量(0)"), length (rest)=2 ("长度（剩余）")) -> (substring=w602:string)
                n229 = String Subset(string=w599, offset (0)=6 ("偏移量(0)"), length (rest)=2 ("长度（剩余）")) -> (substring=w604:string)
                n230 = String Subset(string=w599, offset (0)=0 ("偏移量(0)"), length (rest)=2 ("长度（剩余）")) -> (substring=w596:string)
                n231 = String Subset(string=w599, offset (0)=2 ("偏移量(0)"), length (rest)=2 ("长度（剩余）")) -> (substring=w600:string)
                n232 = Concatenate Strings(w604, " " ("字符串"), w602, " " ("字符串"), w600, " " ("字符串"), w596) -> (w598:string)
              }
            }
            n233 = Search and Replace String(input string="23 F0 20 03 01 00 00 00" ("Data 3"), search string="01 00 00 00" ("Data 5"), replace string=w502, offset=4 ("偏移量(0)")) -> (result string=w509:string)  [unwired: 4 in, 3 out]
            n234 = call "Demo_MakeData.vi"("DataString"=w509) -> ("Data"=w505:u8[], "DataLen"=w520:u8)  [unwired: 9 out]
            n235 = Bundle By Name(cluster=T1 {"ID"=0, "TimeStamp"=0, "TimeFlag"=0, "SendType"=0, "RemoteFlag"=0, "ExternFlag"=0, "DataLen"=0, "Data"=[], "Reserved"=[]} ("Send"), "ID"=w506, "TimeStamp"=u32 0, "TimeFlag"=u8 0, "SendType"=u8 0, "RemoteFlag"=u8 0, "ExternFlag"=u8 0, "DataLen"=w520, "Data"=w505, "Reserved"=u8[] []) -> (w522:T1)
            n236 = Build Array(w522) -> (w521:T1[])
            n237 = call "VCI_Transmit.vi"("Buffer"=w521, "CANIndex"=u32 0, "DevIndex"=u32 0, "DevType"=w514) -> ()  [unwired: 6 in, 2 out]
          }
          event "位置环的kdread": Value Change {
            n238 = event-data() -> ()  [unwired: 1 in, 6 out]
            n239 = stacked-sequence {
              frame #0 {
                (unwired) u32 0 ("CANIndex")
                w619 = T8 4 items=["USB-CAN"=3, "USB-CAN2"=4] ("DevType")
                n240 = local read "ID"() -> (w614:u32)
                n241 = call "Demo_MakeData.vi"("DataString"="40 F0 20 03 00 00 00 00" ("Data 7")) -> ("Data"=w625:u8[], "DataLen"=w626:u8)  [unwired: 9 out]
                n242 = Bundle By Name(cluster=T1 {"ID"=0, "TimeStamp"=0, "TimeFlag"=0, "SendType"=0, "RemoteFlag"=0, "ExternFlag"=0, "DataLen"=0, "Data"=[], "Reserved"=[]} ("Send"), "ID"=w614, "TimeStamp"=u32 0, "TimeFlag"=u8 0, "SendType"=u8 0, "RemoteFlag"=u8 0, "ExternFlag"=u8 0, "DataLen"=w626, "Data"=w625, "Reserved"=u8[] []) -> (w628:T1)
                n243 = Build Array(w628) -> (w627:T1[])
                n244 = call "VCI_Transmit.vi"("Buffer"=w627, "CANIndex"=u32 0, "DevIndex"=u32 0, "DevType"=w619) -> ()  [unwired: 6 in, 2 out]
              }
              frame #1 {
                w629 = T8 4 items=["USB-CAN"=3, "USB-CAN2"=4] ("DevType")
                n245 = Wait (ms)(milliseconds to wait=u32 100 ("等待时间（毫秒）")) -> ()  [unwired: 1 out]
                n246 = call "VCI_Receive.vi"("Len"="Len 4", "CANIndex"=u32 0, "DevIndex"=u32 0, "DevType"=w629) -> ("Recieve"=→"Recieve 4":T1[])  [unwired: 6 in, 1 out]
              }
              frame #2 {
                n247 = local read "Recieve 4"() -> (w651:T1[])
                n248 = Array To Cluster(array=w651) -> (cluster=w650:T13)
                n249 = Unbundle By Name(w650) -> ("Recieve 4[0].Data"=w649:u8[])
                n250 = Array To Cluster(array=w649) -> (cluster=w648:T10)
                n251 = Unbundle By Name(w648) -> ("Data[6]"=w643:u8)
                n252 = Unbundle By Name(w648) -> ("Data[7]"=w642:u8)
                n253 = Unbundle By Name(w648) -> ("Data[5]"=w647:u8)
                n254 = Unbundle By Name(w648) -> ("Data[4]"=w644:u8)
                n255 = Multiply(x=w642, y=16777216) -> (x*y=w638:i32)
                n256 = Multiply(x=w643, y=65536) -> (x*y=w639:i32)
                n257 = Multiply(x=w647, y=256.0) -> (x*y=w645:dbl)
                n258 = Add(x=w644, y=w645) -> (x+y=w637:dbl)
                n259 = Add(x=w639, y=w638) -> (x+y=w636:i32)
                n260 = Add(x=w637, y=w636) -> (x+y=w635:dbl)
                n261 = local write "位置环kd的值"(w635) -> ()
              }
            }
          }
        }
      }
      frame #4 {
      }
      frame #5 {
      }
      frame #6 {
      }
      frame #7 {
      }
    }
  }
